vi "FG Server Instances.vi"(7 "action":T2, 8 "error in":errorcluster, 10 "server refnum in":refnum<vi>, 11 "port":u16) -> (0 "error out":errorcluster, 1 "failed?":bool, 2 "all instances":T1[](array[typedef]), 3 "server instance":T1)   [LabVIEW 2010, in "NI_CCC.lvlib"]
uses:
  NI_CCC.lvlib
  FG Server Instances Action.ctl
  Server Instance Data.ctl
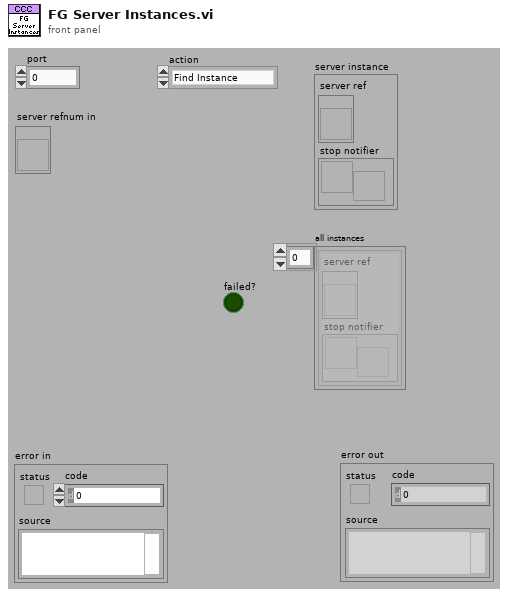
[diagram p1: front panel]
types:
  T1 = typedef "NI_CCC.lvlib/Server Instance Data.ctl" = cluster{"server ref":refnum<vi>, "stop notifier":refnum<notifier>}
  T2 = typedef "NI_CCC.lvlib/FG Server Instances Action.ctl" = enum16{"Find Instance", "Find All", "Register Instance", "Unregister Instance", "Unregister All"}
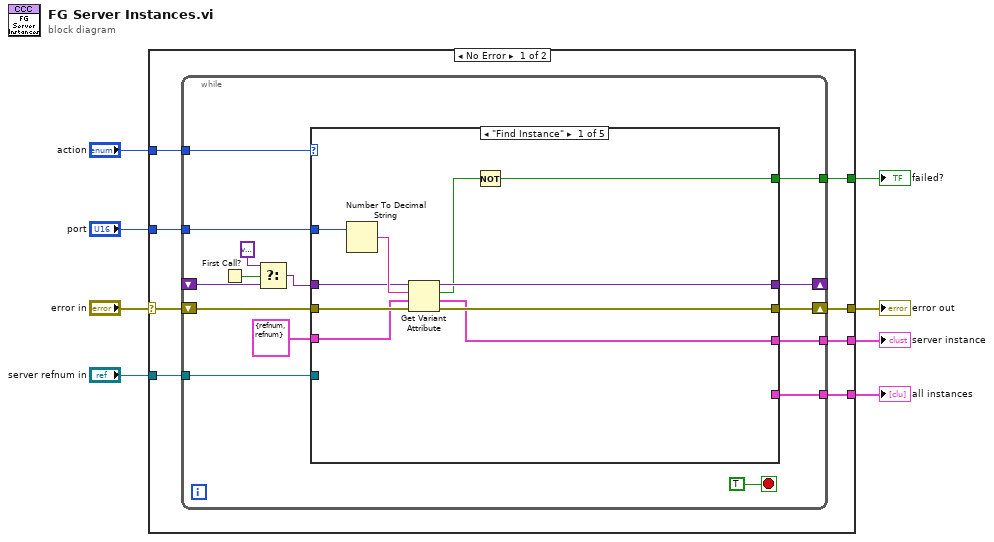
[diagram p0: block diagram]
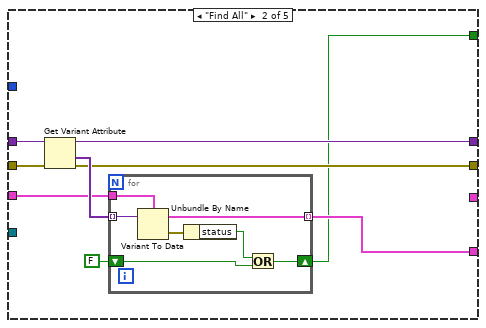
[diagram p2: hidden frame]
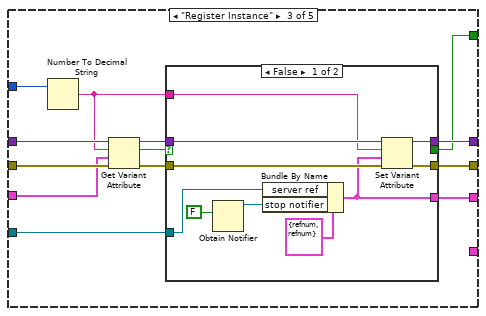
[diagram p3: hidden frame]
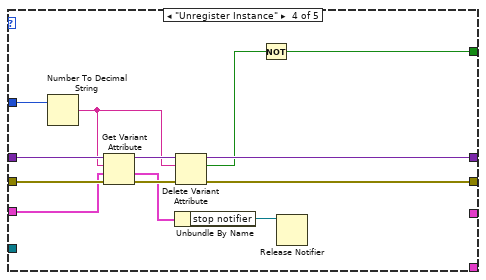
[diagram p5: hidden frame]
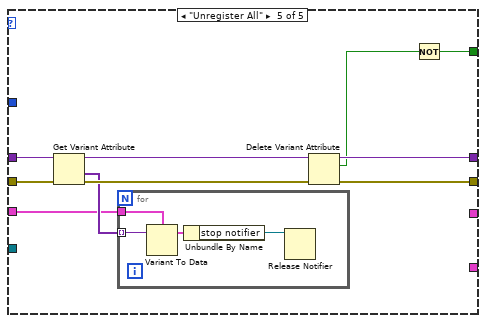
[diagram p6: hidden frame]
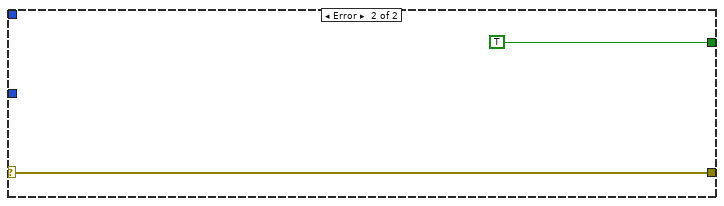
[diagram p7: hidden frame]
diagram:
  n1 = case shown="No Error" "error in" {
    selector: "error in" -> [w13 w111]
    tunnel: "action" -> [w16 _]
    tunnel: "port" -> [w15 _]
    tunnel: "server refnum in" -> [w14 _]
    tunnel: [w12 w111] -> w4
    tunnel: [w11 TRUE] -> w3
    tunnel: [w10 _] -> w2
    tunnel: [w9 _] -> w1
    frame No Error {
      n2 = while {
        tunnel: w16 -> [w30]
        tunnel: w15 -> [w29]
        tunnel: w14 -> [w28]
        shift-right: [w27] -> _
        shift-left: _ -> [w23]
        shift-right: [w25] -> w12
        shift-left: w13 -> [w26]
        tunnel: [w20] -> w11
        tunnel: [w18] -> w10
        tunnel: [w17] -> w9
        stop <- TRUE stop-if-true
        n3 = First Call?() -> (First Call?: T/F=w24:bool)
        n4 = Select(t=variant, s=w24, f=w23) -> (s? t:f=w22:variant)
        n5 = case shown="\"Find Instance\"" w30 {
          tunnel: w29 -> [w41 _ w70 w96 _]
          tunnel: w28 -> [_ _ w60 _ _]
          tunnel: [w39 w46 w63 w94 w106] -> w27
          tunnel: w22 -> [w38 w49 w69 w91 w102]
          tunnel: w26 -> [w37 w48 w68 w89 w100]
          tunnel: [w36 w45 w62 w95 w105] -> w25
          tunnel: T1 {"server ref"=refnum, "stop notifier"=refnum} ("data") -> [w35 w47 w67 w86 w97]
          tunnel: [w33 w42 w59 w92 w103] -> w20
          tunnel: [w32 _ w58 _ _] -> w18
          tunnel: [_ w44 _ _ _] -> w17
          frame "Find Instance" {
            n6 = Number To Decimal String(number=w41) -> (decimal integer string=w40:string)  [unwired: 1 in]
            n7 = Get Variant Attribute(Variant=w38, name=w40, default value (empty Variant)=w35, error in=w37) -> (duplicate Variant=w39:variant, found=w34:bool, value=w32:T1, error out=w36:errorcluster)
            n8 = Not(x=w34) -> (.not. x?=w33:bool)
          }
          frame "Find All" {
            n9 = Get Variant Attribute(Variant=w49, error in=w48) -> (duplicate Variant=w46:variant, values=w50:variant[], error out=w45:errorcluster)  [unwired: 2 in, 1 out]
            n10 = for {
              tunnel: w50 -> [w57] mode=indexing
              tunnel: w47 -> [w56]
              tunnel: [w55] -> w44 mode=indexing
              shift-right: [w52] -> w42
              shift-left: FALSE -> [w51]
              n11 = Variant To Data(Variant=w57, type=w56) -> (error out=w54:errorcluster, data=w55:T1)  [unwired: 1 in]
              n12 = Unbundle By Name(w54) -> ("status"=w53:bool)
              n13 = Or(x=w53, y=w51) -> (x .or. y?=w52:bool)
            }
          }
          frame "Register Instance" {
            n14 = Number To Decimal String(number=w70) -> (decimal integer string=w64:string)  [unwired: 1 in]
            n15 = Get Variant Attribute(Variant=w69, name=w64, default value (empty Variant)=w67, error in=w68) -> (duplicate Variant=w65:variant, found=w61:bool, error out=w66:errorcluster)  [unwired: 1 out]
            n16 = case shown="False" w61 {
              selector: w61 -> [_ w81]
              tunnel: w66 -> [w79 w82]
              tunnel: w65 -> [w80 w83]
              tunnel: w64 -> [w78 _]
              tunnel: w60 -> [w73 _]
              tunnel: [w77 w83] -> w63
              tunnel: [w76 w82] -> w62
              tunnel: [_ w81] -> w59
              tunnel: [w71 _] -> w58
              frame False {
                n17 = Obtain Notifier(notification data type=FALSE) -> (notifier out=w72:refnum<notifier>)  [unwired: 3 in, 2 out]
                n18 = Bundle By Name(cluster=T1 {"server ref"=refnum, "stop notifier"=refnum} ("data"), "server ref"=w73, "stop notifier"=w72) -> (w71:T1)
                n19 = Set Variant Attribute(Variant=w80, name=w78, value=w71, error in=w79) -> (Variant out=w77:variant, error out=w76:errorcluster)  [unwired: 1 out]
              }
              frame True {
              }
            }
          }
          frame "Unregister Instance" {
            n20 = Number To Decimal String(number=w96) -> (decimal integer string=w87:string)  [unwired: 1 in]
            n21 = Get Variant Attribute(Variant=w91, name=w87, default value (empty Variant)=w86, error in=w89) -> (duplicate Variant=w90:variant, value=w85:T1, error out=w88:errorcluster)  [unwired: 1 out]
            n22 = Unbundle By Name(w85) -> ("stop notifier"=w84:refnum<notifier>)
            n23 = Delete Variant Attribute(4:w88, 6:w87, 7:w90) -> (0:w95:errorcluster, 2:w93:bool, 3:w94:variant)
            n24 = Not(x=w93) -> (.not. x?=w92:bool)
            n25 = Release Notifier(notifier=w84) -> ()  [unwired: 2 in, 3 out]
          }
          frame "Unregister All" {
            n26 = Get Variant Attribute(Variant=w102, error in=w100) -> (duplicate Variant=w101:variant, values=w98:variant[], error out=w99:errorcluster)  [unwired: 2 in, 1 out]
            n27 = for {
              tunnel: w98 -> [w110] mode=indexing
              tunnel: w97 -> [w109]
              n28 = Variant To Data(Variant=w110, type=w109) -> (data=w108:T1)  [unwired: 1 in, 1 out]
              n29 = Unbundle By Name(w108) -> ("stop notifier"=w107:refnum<notifier>)
              n30 = Release Notifier(notifier=w107) -> ()  [unwired: 2 in, 3 out]
            }
            n31 = Delete Variant Attribute(4:w99, 7:w101) -> (0:w105:errorcluster, 2:w104:bool, 3:w106:variant)  [unwired: 1 in]
            n32 = Not(x=w104) -> (.not. x?=w103:bool)
          }
        }
      }
    }
    frame Error {
    }
  }
  "error out" <- w4
  "failed?" <- w3
  "server instance" <- w2
  "all instances" <- w1
